vi "str2code.vi"(2 "错误输入":errorcluster, 3 "input":string) -> (0 "error out":errorcluster caption="error IO", 1 "Output":T1)   [LabVIEW 2012]
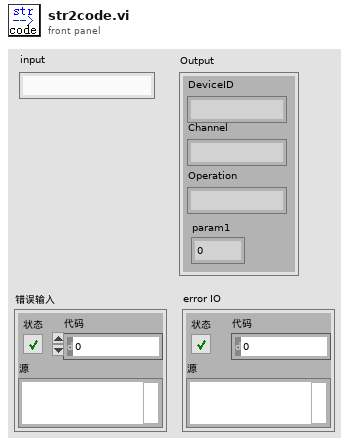
[diagram p1: front panel]
types:
  T1 = cluster{"DeviceID":string, "Channel":string, "param1":dbl, "Operation":string}
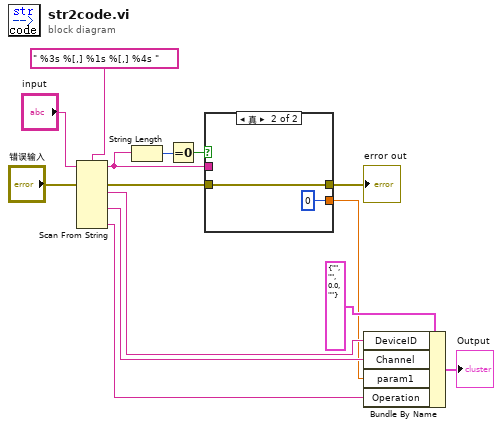
[diagram p0: block diagram]
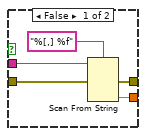
[diagram p2: hidden frame]
diagram:
  n1 = Scan From String(format string=" %3s %[,] %1s %[,] %4s " ("格式字符串"), input string="input", error in="错误输入") -> (remaining string=w5:string, error out=w3:errorcluster, output 1=w10:string, output 3=w9:string, output 5=w7:string)  [unwired: 8 in, 1 out]
  n2 = String Length(string=w5) -> (length=w8:i32)
  n3 = Equal To 0?(x=w8) -> (x = 0?=w6:bool)
  n4 = case shown="真" w6 {
    tunnel: w5 -> [w19 _]
    tunnel: [w17 0] -> w4
    tunnel: w3 -> [w16 w20]
    tunnel: [w15 w20] -> w2
    frame False {
      n5 = Scan From String(format string="%[,] %f" ("格式字符串"), input string=w19, error in=w16) -> (error out=w15:errorcluster, output 2=w17:dbl)  [unwired: 4 in, 2 out]
    }
    frame True {
    }
  }
  "error out" <- w2
  n6 = Bundle By Name(cluster=T1 {"DeviceID"="", "Channel"="", "param1"=0.0, "Operation"=""} ("Output"), "DeviceID"=w10, "Channel"=w9, "param1"=w4, "Operation"=w7) -> (→"Output":T1)
